vi "Write RDS Router Enqeuer.vi"(8 "error in (no error)":errorcluster, 10 "RDS Router Enqueuer":refnum<class "Message Enqueuer.lvclass">, 11 "RDS Child Actor in":refnum<class "RDS Parent Actor.lvclass">) -> (0 "error out":errorcluster, 3 "RDS Child Actor out":refnum<class "RDS Parent Actor.lvclass">)   [LabVIEW 2015, in "RDS Abstracts.lvlib" / "RDS Parent Actor.lvlib" / "RDS Parent Actor.lvclass"]
uses:
  RDS Parent Actor.lvclass
  <vilib>/ActorFramework/Message Enqueuer/Message Enqueuer.lvclass
  RDS Parent Actor.lvclass/RDS Parent Actor.ctl
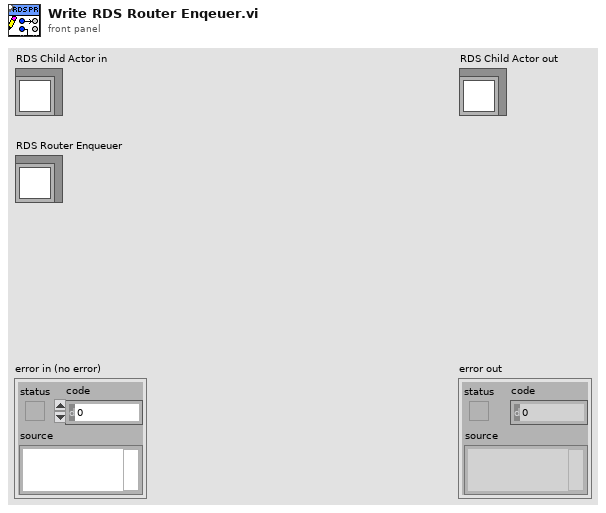
[diagram p1: front panel]
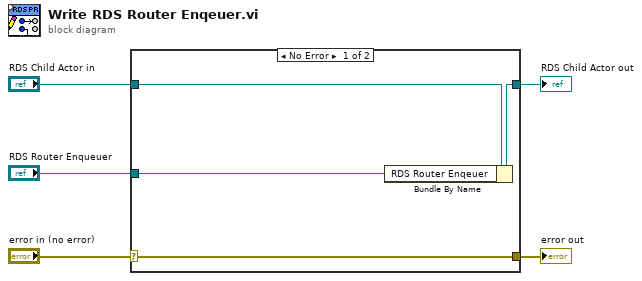
[diagram p0: block diagram]
diagram:
  n1 = case shown="No Error" "error in (no error)" {
    selector: "error in (no error)" -> [w9 w10]
    tunnel: [w9 w10] -> w4
    tunnel: [w7 w11] -> w2
    tunnel: "RDS Child Actor in" -> [w8 w11]
    tunnel: "RDS Router Enqueuer" -> [w6 _]
    frame No Error {
      n2 = Bundle By Name(cluster=w8, "RDS Router Enqeuer"=w6) -> (w7:refnum<class "RDS Parent Actor.lvclass">)
    }
    frame Error {
    }
  }
  "error out" <- w4
  "RDS Child Actor out" <- w2
